vi "Calibrate_Sums_orig.vi"(8 "error in (no error)":errorcluster, 11 "Signal Channel":enum16{"Red", "Green"}(ring)) -> (0 "error out":errorcluster, 2 "sum":dbl)   [LabVIEW 2020]
doc: "Use this template to create a dialog box with event handling."
uses:
  Globals/gl_Calibration globals.vi
  Typedefs/Top level VI states.ctl
  Global Variables/gl_Images.vi
  Global Variables/General Globals.vi
  TypeDefs/Control Plane.ctl
panel:
  out "Objects found":T1(array[cluster])
  in  "Shape Adapted Options in":T2={"Number of Histogram Bins"=8, "Blending Parameter (%)"=10.0, "Max Scale Change (%)"=1.0, "Max Rotation Change"=40.0, "Max Shape Change (%)"=1.0, "Maximum Iterations"=15}
  out "Distance Array (Y)":dbl[][](array[numeric])
  in  "Delay 3":u32=1000
  out "Image 2":T3(plugin-control)
  out "Distance Array (X)":dbl[][](array[numeric])
  out "Image":T3(plugin-control)
  in  "Range":cluster{"Lower value":sgl, "Upper value":sgl}={"Lower value"=40.0, "Upper value"=255.0}
  in  "Delay 2":u32=1000
  in  "Delay":u32=1000
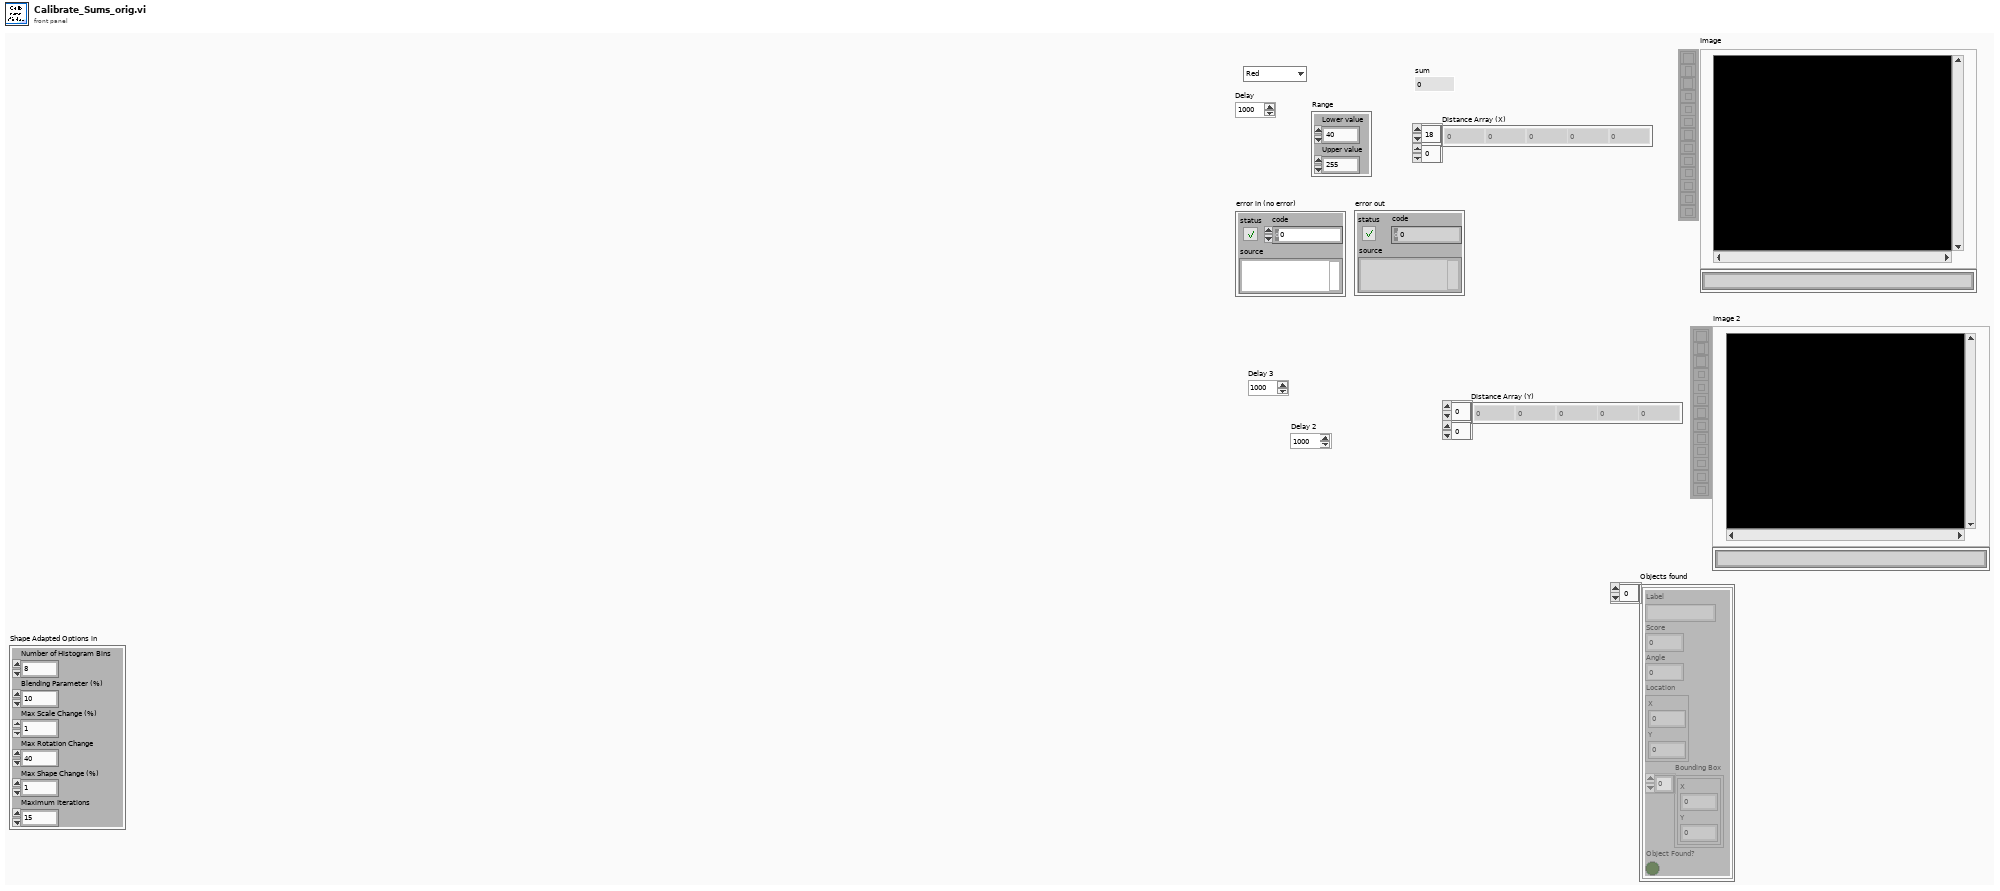
[diagram p1: front panel]
types:
  T1 = cluster{"Label":string, "Score":i32, "Angle":dbl, "Location":cluster{"X":dbl, "Y":dbl}, "Bounding Box":cluster{"X":dbl, "Y":dbl}[], "Object Found?":bool}[]
  T2 = cluster{"Number of Histogram Bins":i32, "Blending Parameter (%)":dbl, "Max Scale Change (%)":dbl, "Max Rotation Change":dbl, "Max Shape Change (%)":dbl, "Maximum Iterations":i32}
  T3 = typedef "IMAQ Image.ctl" = refnum<image>
  T4 = enum16{"Create tracking", "Setup Object", "Track Object", "Close"}
  T5 = enum16{"Raster", "Structural", "Pointing", "Mini Scan", "Alignment"}
  T6 = typedef "Top level VI states.ctl" = enum16{"None", "Initialise UI", "<STACK PROTOCOL STATES>", "AOL Zstack-START", "AOL Zstack-STOP", "Motor Zstack-START", "Motor Zstack-STOP", "<ACQUISITION PROTOCOL STATES> ", "Functional Acquisition-START", "Functional Acquisition-STOP", "Single Plane Acquisition-START", "Single Plane Acquisition-STOP", "Volume Acquisition-START", "Volume Acquisition-STOP", "<LIVE IMAGING PROTOCOL STATES>", "Live Imaging-START", "Live Imaging-STOP", "Live Plane Imaging-START", "Live Plane Imaging-STOP", "Live Volume Imaging-START", "Live Volume Imaging-STOP", "<MOVEMENT CORRECTION PROTOCOL STATES>", "EXIT"}
  T7 = typedef "Control Plane.ctl" = enum16{"XY-X", "XY-Y", "Z"}
  T8 = typedef "IMAQ Rectangle" = cluster{"Left":i32, "Top":i32, "Right":i32, "Bottom":i32, "Rotation":dbl}
  T9 = typedef "General Scan Parameters.ctl" = cluster{"Field of View":sgl, "Frame Size":u16, "Dwell Time (ms)":dbl, "Wavelength (nm)":dbl, "Zoom":dbl, "AOL Xc":sgl, "AOL Yc":sgl, "AOL Zc":sgl, "AOL Mode":enum16{"Raster", "Structural", "Pointing", "Mini Scan", "Alignment"}, "Imaging Mode":enum16{"Live Imaging", "AOL Zstack", "Motor Zstack", "Functional Imaging"}}
  T10 = cluster{"Particle Measurements (Pixels)[0]":dbl, "Particle Measurements (Pixels)[1]":dbl}[]
  T11 = typedef "Current Calibration Parameters.ctl" = cluster{"Sum X":dbl, "Sum Y":dbl, "Diff X":dbl, "Diff Y":dbl, "Distortion Correction":dbl, "Z_norm to um_scaling":dbl, "X_norm to um_scaling":dbl, "Samples to Wait after Trigger":dbl, "Slip Cycle":dbl}
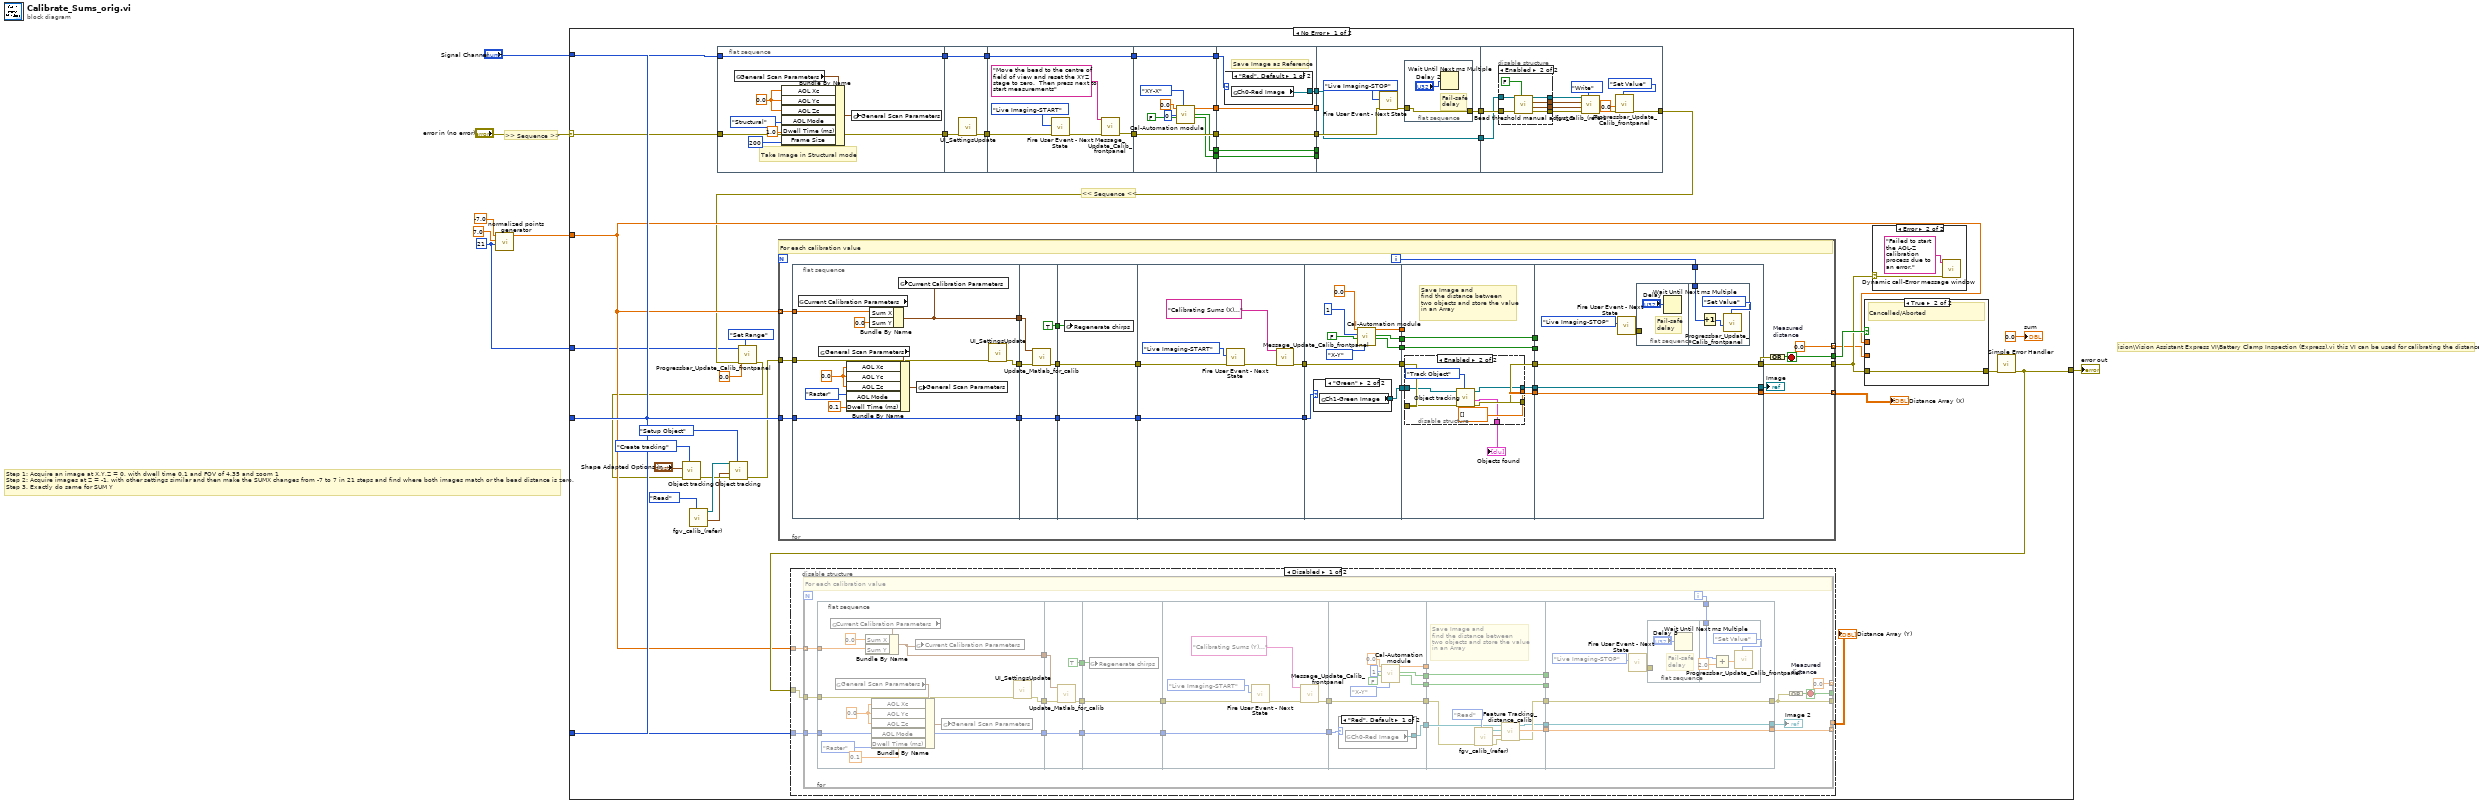
[diagram p0: block diagram]
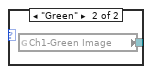
[diagram p2: hidden frame]
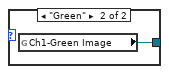
[diagram p4: hidden frame]
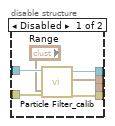
[diagram p5: hidden frame]
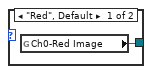
[diagram p6: hidden frame]
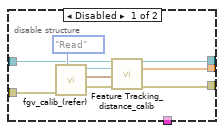
[diagram p7: hidden frame]
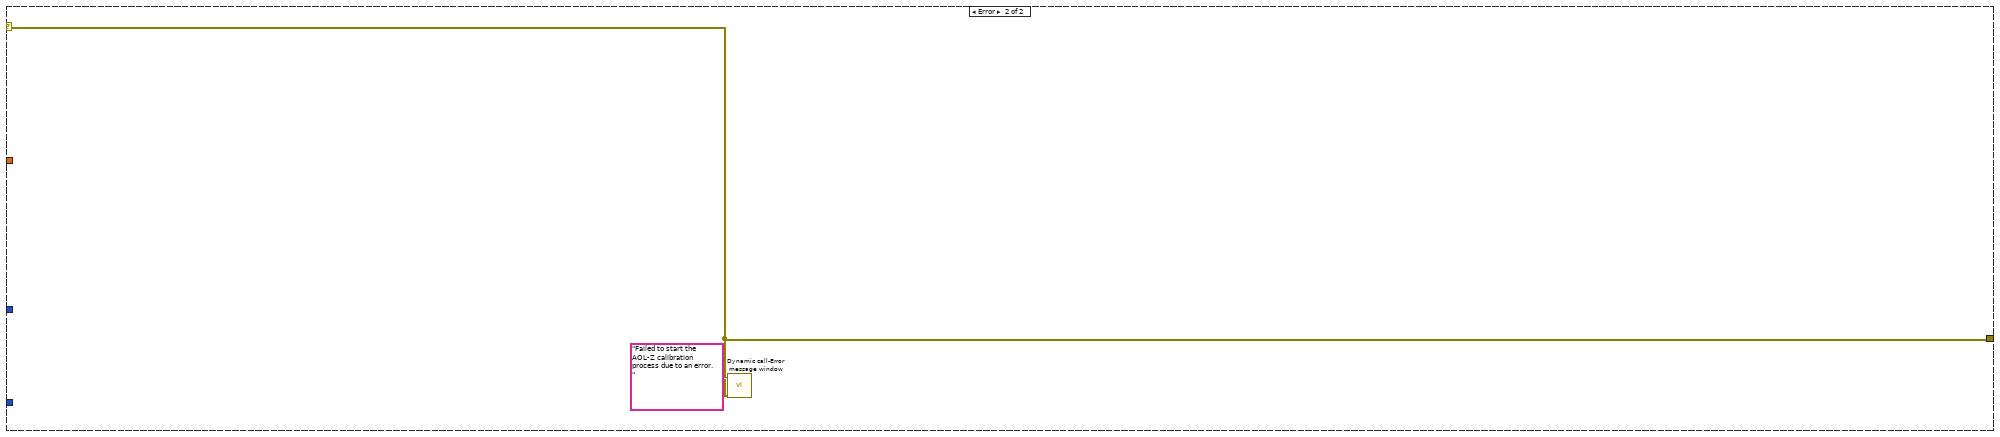
[diagram p10: hidden frame]
diagram:
  w1 = 21 ("number of points")
  # ">> Sequence >>"
  # "ision\\Vision Assistant Express VI\\Battery Clamp Inspection (Express).vi this VI can be used for calibrating the distance"
  # "Step 1: Acquire an image at X,Y,Z = 0, with dwell time 0.1 and FOV of 4.35 and zoom 1\nStep 2: Acquire images at Z = -1, with other settings similar and then make the SUMX changes from -7 to 7 in 21 steps and find where both images match or the bead distance is zero.\nStep 3. Exactly do same for SUM Y"
  n1 = call "normalized points generator.vi"("number of points"=w1, "maximum"=7.0, "minimum"=-7.0) -> ("normalised array"=w5:dbl[])  [unwired: 7 in, 1 out]
  n2 = case shown="No Error" "error in (no error)" {
    selector: "error in (no error)" -> [w45 w314]
    tunnel: w5 -> [w22 _]
    tunnel: [w23 w314] -> w7
    tunnel: "Signal Channel" -> [w27 _]
    tunnel: "Signal Channel" -> [w29 _]
    tunnel: "Signal Channel" -> [w24 _]
    tunnel: w1 -> [w17 _]
    frame No Error {
      # "<< Sequence <<"
      n3 = call "fgv_calib_(refer).vi"("State"=enum16{"Write", "Read"}."Read") -> ("enclosure box OUT"=w10:T8, "Reference Image"=w12:T3)  [unwired: 7 in, 2 out]
      n4 = flat-sequence {
        tunnel: w45 -> [w149]
        tunnel: [w149] -> w46
        tunnel: [w148] -> w30
        tunnel: w29 -> [w148]
        tunnel: [w155] -> w48
        tunnel: w46 -> [w154]
        tunnel: [w153] -> w31
        tunnel: w30 -> [w153]
        tunnel: [w160] -> w47
        tunnel: w48 -> [w161]
        tunnel: [w156] -> w32
        tunnel: w31 -> [w156]
        tunnel: [w169] -> w37
        tunnel: [w170] -> w39
        tunnel: w47 -> [w170]
        tunnel: [w165] -> w41
        tunnel: [w166] -> w43
        tunnel: [w163] -> w33
        tunnel: w32 -> [w163]
        tunnel: w43 -> [w176]
        tunnel: [w176] -> w42
        tunnel: w41 -> [w175]
        tunnel: [w175] -> w40
        tunnel: w39 -> [w174]
        tunnel: [w174] -> w38
        tunnel: w37 -> [w171]
        tunnel: [w171] -> w36
        tunnel: w33 -> [w173]
        tunnel: [w172] -> w28
        tunnel: w42 -> [_]
        tunnel: w40 -> [_]
        tunnel: w38 -> [w181]
        tunnel: w36 -> [_]
        tunnel: [w180] -> w35
        tunnel: w28 -> [w179]
        tunnel: [w179] -> w26
        tunnel: [w188] -> w18
        tunnel: w35 -> [w196]
        tunnel: w26 -> [w191]
        frame #0 {
          w150 = sgl 0.0 ("AOL Yc")
          # "Take Image in Structural mode"
          n5 = global read "gl_Calibration globals.vi" "General Scan Parameters"() -> (w152:T9)
          n6 = Bundle By Name(cluster=w152, "AOL Xc"=w150, "AOL Yc"=w150, "AOL Zc"=w150, "AOL Mode"=T5."Structural", "Dwell Time (ms)"=1.0, "Frame Size"=u16 200) -> (w151:T9)
          n7 = global write "gl_Calibration globals.vi" "General Scan Parameters"(w151) -> ()
        }
        frame #1 {
          n8 = call "UI_SettingsUpdate.vi"("error in (no error)"=w154) -> ("error out"=w155:errorcluster)  [unwired: 10 in]
        }
        frame #2 {
          n9 = call "Fire User Event - Next State.vi"("Error In"=w161, "\"UI Handler loop\" case to execute"=Top_level_VI_states."Live Imaging-START" ("\"UI Handler loop\" case to execute")) -> ("Error Out"=w159:errorcluster)  [unwired: 9 in]
          n10 = call "Message_Update_Calib_frontpanel.vi"("error in (no error)"=w159, "Message"="Move the bead to the centre of field of view and reset the XYZ stage to zero.  Then press next to start measurements") -> ("error out"=w160:errorcluster)  [unwired: 9 in]
        }
        frame #3 {
          n11 = call "Cal-Automation module.vi"("Parameter"=Control_Plane."XY-X", "Timed out while waiting for acknowledgement in"=FALSE, "FOR loop index"=0, "Initial motor position (um)"=sgl 0.0) -> ("Motor timed out or errored out"=w165:bool, "Cancelled"=w166:bool, "Measured cal value"=w169:sgl)  [unwired: 4 in, 1 out]
        }
        frame #4 {
          # "Save Image as Reference"
          n12 = case shown="\"Red\", Default" w173 {
            tunnel: [w177 w178] -> w172
            frame "Red", Default {
              n13 = global read "gl_Images.vi" "Ch0-Red Image"() -> (w177:T3)
            }
            frame "Green" {
              n14 = global read "gl_Images.vi" "Ch1-Green Image"() -> (w178:T3)
            }
          }
        }
        frame #5 {
          n15 = call "Fire User Event - Next State.vi"("Error In"=w181, "\"UI Handler loop\" case to execute"=Top_level_VI_states."Live Imaging-STOP" ("\"UI Handler loop\" case to execute")) -> ("Error Out"=w183:errorcluster)  [unwired: 9 in]
          n16 = flat-sequence {
            tunnel: w183 -> [w184]
            tunnel: [w184] -> w180
            frame #0 {
              # "Fail-safe delay"
              n17 = Wait Until Next ms Multiple(millisecond multiple="Delay 2") -> ()  [unwired: 1 out]
            }
          }
        }
        frame #6 {
          n18 = disable-structure shown="Enabled" {
            disable-tunnel: w196 -> [w202 w209]
            disable-tunnel: [w201 w206] -> w195
            disable-tunnel: [w200 w205] -> w194
            disable-tunnel: [w199 w204] -> w193
            disable-tunnel: w191 -> [w198 w208]
            disable-tunnel: [_ w203] -> w186
            frame Disabled {
              n19 = call "Particle Filter_calib.vi"("Range"="Range", "error in"=w202, "Source Image"=w198) -> ("error out"=w201:errorcluster, "Location in Pixels"=w199:T10, "Ref Image (8 bit)"=w200:T3)  [unwired: 6 in]
            }
            frame Enabled {
              n20 = call "Bead threshold manual adjust 2.vi"("Standalone(F)"=FALSE, "error in (no error)"=w209, "Image In"=w208) -> ("error out"=w206:errorcluster, "enclosure box"=w203:T8, "Centroid array"=w204:T10, "Source Image"=w205:T3)  [unwired: 4 in]
            }
          }
          n21 = call "fgv_calib_(refer).vi"("State"=enum16{"Write", "Read"}."Write", "error in (no error)"=w195, "enclosure box IN"=w186, "Location in Pixels"=w193, "Reference Image"=w194) -> ("error in (no error)"=w189:errorcluster)  [unwired: 3 in, 3 out]
          n22 = call "Progressbar_Update_Calib_frontpanel.vi"("Ops"=enum16{"Set Value", "Set Range"}."Set Value", "error in (no error)"=w189, "Value"=0.0) -> ("error out"=w188:errorcluster)  [unwired: 8 in]
        }
      }
      n23 = call "Progressbar_Update_Calib_frontpanel.vi"("Ops"=enum16{"Set Value", "Set Range"}."Set Range", "error in (no error)"=w18, "Scale.Range:Minimum"=0.0, "Scale.Range:Maximum"=w17) -> ("error out"=w9:errorcluster)  [unwired: 7 in]
      n24 = call "Object tracking.vi"("Tracking Ops"=T4."Create tracking", "error in (no error)"=w9, "Shape Adapted Options in"="Shape Adapted Options in") -> ("error out"=w11:errorcluster)  [unwired: 2 in, 6 out]
      n25 = call "Object tracking.vi"("Tracking Ops"=T4."Setup Object", "error in (no error)"=w11, "Rectangle"=w10, "Image IN"=w12) -> ("error out"=w8:errorcluster)  [unwired: 1 in, 6 out]
      n26 = for {
        tunnel: w22 -> [w238] mode=indexing
        tunnel: [w233] -> w50
        tunnel: [w234] -> w49
        tunnel: w8 -> [w236]
        tunnel: [w224] -> w44 mode=indexing
        tunnel: w27 -> [w223]
        tunnel: [w218] -> w25 mode=indexing
        i -> [w210]
        stop <- w233 stop-if-true
        w224 = sgl 0.0  # Measured  distance
        # "For each calibration value"
        n27 = flat-sequence {
          tunnel: w238 -> [w249]
          tunnel: w236 -> [w240]
          tunnel: [w239] -> w235
          tunnel: [w248] -> w225
          tunnel: w223 -> [w246]
          tunnel: [w246] -> w222
          tunnel: w235 -> [w255]
          tunnel: [w254] -> w217
          tunnel: w225 -> [w253]
          tunnel: w222 -> [w252]
          tunnel: [w252] -> w215
          tunnel: [TRUE] -> w213
          tunnel: w217 -> [w258]
          tunnel: [w258] -> w216
          tunnel: w215 -> [w257]
          tunnel: [w257] -> w214
          tunnel: w213 -> [w256]
          tunnel: [w263] -> w237
          tunnel: w216 -> [w264]
          tunnel: w214 -> [w259]
          tunnel: [w259] -> w221
          tunnel: [w273] -> w232
          tunnel: [w274] -> w231
          tunnel: w237 -> [w274]
          tunnel: [w269] -> w229
          tunnel: [w270] -> w227
          tunnel: w221 -> [w265]
          tunnel: [w266] -> w220
          tunnel: w232 -> [_]
          tunnel: w231 -> [w280]
          tunnel: [w279] -> w230
          tunnel: w229 -> [w284]
          tunnel: [w284] -> w228
          tunnel: w227 -> [w283]
          tunnel: [w283] -> w226
          tunnel: w220 -> [w282]
          tunnel: [w281] -> w219
          tunnel: [w278] -> w212
          tunnel: w230 -> [w305]
          tunnel: [w305] -> w234
          tunnel: w228 -> [_]
          tunnel: w226 -> [_]
          tunnel: w219 -> [w303]
          tunnel: [w303] -> w218
          tunnel: [w302] -> w211
          tunnel: w212 -> [w302]
          tunnel: w210 -> [w301]
          frame #0 {
            w243 = sgl 0.0 ("AOL Yc")
            n28 = global read "gl_Calibration globals.vi" "Current Calibration Parameters"() -> (w250:T11)
            n29 = global read "gl_Calibration globals.vi" "General Scan Parameters"() -> (w245:T9)
            n30 = Bundle By Name(cluster=w245, "AOL Xc"=w243, "AOL Yc"=w243, "AOL Zc"=w243, "AOL Mode"=T5."Raster", "Dwell Time (ms)"=0.1) -> (w244:T9)
            n31 = Bundle By Name(cluster=w250, "Sum X"=w249, "Sum Y"=0.0) -> (w248:T11)
            n32 = global write "gl_Calibration globals.vi" "Current Calibration Parameters"(w248) -> ()
            n33 = global write "gl_Calibration globals.vi" "General Scan Parameters"(w244) -> ()
            n34 = call "UI_SettingsUpdate.vi"("error in (no error)"=w240) -> ("error out"=w239:errorcluster)  [unwired: 10 in]
          }
          frame #1 {
            n35 = call "Update_Matlab_for_calib.vi"("error in (no error)"=w255, "Current Calibration Parameters"=w253) -> ("error out"=w254:errorcluster)  [unwired: 9 in]
          }
          frame #2 {
            n36 = global write "General Globals.vi" "Regenerate chirps"(w256) -> ()
          }
          frame #3 {
            n37 = call "Fire User Event - Next State.vi"("Error In"=w264, "\"UI Handler loop\" case to execute"=Top_level_VI_states."Live Imaging-START" ("\"UI Handler loop\" case to execute")) -> ("Error Out"=w262:errorcluster)  [unwired: 9 in]
            n38 = call "Message_Update_Calib_frontpanel.vi"("error in (no error)"=w262, "Message"="Calibrating Sums (X)...") -> ("error out"=w263:errorcluster)  [unwired: 9 in]
          }
          frame #4 {
            n39 = case shown="\"Green\"" w265 {
              tunnel: [w275 w276] -> w266
              frame "Red", Default {
                n40 = global read "gl_Images.vi" "Ch0-Red Image"() -> (w275:T3)
              }
              frame "Green" {
                n41 = global read "gl_Images.vi" "Ch1-Green Image"() -> (w276:T3)
              }
            }
            n42 = call "Cal-Automation module.vi"(6:enum16{"X-Y", "Z"}."X-Y" ("StageSelection"), "Timed out while waiting for acknowledgement in"=FALSE, "FOR loop index"=1, "Initial motor position (um)"=sgl 0.0) -> ("Motor timed out or errored out"=w269:bool, "Cancelled"=w270:bool, "Measured cal value"=w273:sgl)  [unwired: 4 in, 1 out]
          }
          frame #5 {
            # "Save Image and \nfind the distance between\ntwo objects and store the value\nin an Array"
            n43 = disable-structure shown="Enabled" {
              disable-tunnel: w282 -> [w290 w299]
              disable-tunnel: [w289 dbl[] [] ("Distance Array")] -> w281
              disable-tunnel: w280 -> [w287 w300]
              disable-tunnel: [w286 w295] -> w279
              disable-tunnel: [w285 w296] -> w278
              disable-tunnel: [_ w294] -> w277
              frame Disabled {
                n44 = call "fgv_calib_(refer).vi"("State"=enum16{"Write", "Read"}."Read", "error in (no error)"=w287) -> ("error in (no error)"=w288:errorcluster, "Location in Pixels"=w291:T10, "Reference Image"=w292:T3)  [unwired: 6 in, 1 out]
                n45 = call "Feature Tracking_distance_calib.vi"("Current Image"=w290, "Reference Image"=w292, "Location in Pixels"=w291, "error in (no error)"=w288) -> ("Analysed Image"=w285:T3, "Distance Array"=w289:dbl[], "error out"=w286:errorcluster)  [unwired: 9 in]
              }
              frame Enabled {
                n46 = call "Object tracking.vi"("Tracking Ops"=T4."Track Object", "error in (no error)"=w300, "Image IN"=w299) -> ("error out"=w295:errorcluster, "Objects found"=w294:T1, "Image OUT"=w296:T3)  [unwired: 2 in, 4 out]
              }
            }
            "Objects found" <- w277
          }
          frame #6 {
            n47 = call "Fire User Event - Next State.vi"("\"UI Handler loop\" case to execute"=Top_level_VI_states."Live Imaging-STOP" ("\"UI Handler loop\" case to execute")) -> ("Error Out"=w306:errorcluster)  [unwired: 10 in]
            n48 = flat-sequence {
              tunnel: w306 -> [_]
              tunnel: w301 -> [w309]
              frame #0 {
                # "Fail-safe delay"
                n49 = Wait Until Next ms Multiple(millisecond multiple="Delay") -> ()  [unwired: 1 out]
              }
              frame #1 {
                n50 = Increment(x=w309) -> (x+1=w308:i32)
                n51 = call "Progressbar_Update_Calib_frontpanel.vi"("Ops"=enum16{"Set Value", "Set Range"}."Set Value", "Value"=w308) -> ()  [unwired: 9 in, 1 out]
              }
            }
          }
        }
        n52 = Compound Arithmetic op=OR(w234) -> (w233:bool)
        "Image" <- w211
      }
      "Distance Array (X)" <- w25
      n53 = case shown="True" w50 {
        tunnel: w22 -> [_ _]
        tunnel: w44 -> [_ _]
        tunnel: [_ w313] -> w51
        tunnel: w49 -> [_ w313]
        frame False {
          # "find zero value from the array"
        }
        frame True {
          # "Cancelled/Aborted"
        }
      }
      n54 = case shown="Error" w49 {
        selector: w49 -> [_ w312]
        frame No Error {
        }
        frame Error {
          n55 = call "Dynamic call-Error message window.vi"("error in (no error)"=w312, "Error Message"="Failed to start the AOL-Z calibration process due to an error.") -> ()  [unwired: 9 in, 1 out]
        }
      }
      n56 = call <vilib>:"Simple Error Handler.vi"("error in (no error)"=w51) -> ("error out"=w23:errorcluster)  [unwired: 4 in, 4 out]
      n57 = disable-structure shown="Disabled" {
        disable-tunnel: w24 -> [w55 _]
        disable-tunnel: w23 -> [w54 _]
        disable-tunnel: w22 -> [w53 _]
        disable-tunnel: [w52 _] -> w21
        frame Disabled {
          n58 = for {
            tunnel: w53 -> [w84] mode=indexing
            tunnel: [w79] -> _
            tunnel: [w80] -> _
            tunnel: w54 -> [w82]
            tunnel: [w70] -> _ mode=indexing
            tunnel: w55 -> [w69]
            tunnel: [w64] -> w52 mode=indexing
            i -> [w56]
            stop <- w79 stop-if-true
            w70 = sgl 0.0  # Measured  distance
            # "For each calibration value"
            n59 = flat-sequence {
              tunnel: w84 -> [w85]
              tunnel: w82 -> [w88]
              tunnel: [w87] -> w81
              tunnel: [w95] -> w71
              tunnel: w69 -> [w94]
              tunnel: [w94] -> w68
              tunnel: w81 -> [w101]
              tunnel: [w100] -> w63
              tunnel: w71 -> [w99]
              tunnel: w68 -> [w98]
              tunnel: [w98] -> w61
              tunnel: [TRUE] -> w59
              tunnel: w63 -> [w104]
              tunnel: [w104] -> w62
              tunnel: w61 -> [w103]
              tunnel: [w103] -> w60
              tunnel: w59 -> [w102]
              tunnel: [w109] -> w83
              tunnel: w62 -> [w110]
              tunnel: w60 -> [w105]
              tunnel: [w105] -> w67
              tunnel: [w119] -> w78
              tunnel: [w120] -> w77
              tunnel: w83 -> [w120]
              tunnel: [w115] -> w75
              tunnel: [w116] -> w73
              tunnel: w67 -> [w111]
              tunnel: [w112] -> w66
              tunnel: w78 -> [_]
              tunnel: w77 -> [w125]
              tunnel: [w124] -> w76
              tunnel: w75 -> [w133]
              tunnel: [w133] -> w74
              tunnel: w73 -> [w132]
              tunnel: [w132] -> w72
              tunnel: w66 -> [w128]
              tunnel: [w127] -> w65
              tunnel: [w123] -> w58
              tunnel: w76 -> [w138]
              tunnel: [w138] -> w80
              tunnel: w74 -> [_]
              tunnel: w72 -> [_]
              tunnel: w65 -> [w136]
              tunnel: [w136] -> w64
              tunnel: [w135] -> w57
              tunnel: w58 -> [w135]
              tunnel: w56 -> [w134]
              frame #0 {
                w91 = sgl 0.0 ("AOL Yc")
                n60 = global read "gl_Calibration globals.vi" "Current Calibration Parameters"() -> (w96:T11)
                n61 = global read "gl_Calibration globals.vi" "General Scan Parameters"() -> (w93:T9)
                n62 = Bundle By Name(cluster=w96, "Sum X"=0.0 ("Sum Y"), "Sum Y"=w85) -> (w95:T11)
                n63 = Bundle By Name(cluster=w93, "AOL Xc"=w91, "AOL Yc"=w91, "AOL Zc"=w91, "AOL Mode"=T5."Raster", "Dwell Time (ms)"=0.1) -> (w92:T9)
                n64 = global write "gl_Calibration globals.vi" "Current Calibration Parameters"(w95) -> ()
                n65 = global write "gl_Calibration globals.vi" "General Scan Parameters"(w92) -> ()
                n66 = call "UI_SettingsUpdate.vi"("error in (no error)"=w88) -> ("error out"=w87:errorcluster)  [unwired: 10 in]
              }
              frame #1 {
                n67 = call "Update_Matlab_for_calib.vi"("error in (no error)"=w101, "Current Calibration Parameters"=w99) -> ("error out"=w100:errorcluster)  [unwired: 9 in]
              }
              frame #2 {
                n68 = global write "General Globals.vi" "Regenerate chirps"(w102) -> ()
              }
              frame #3 {
                n69 = call "Fire User Event - Next State.vi"("Error In"=w110, "\"UI Handler loop\" case to execute"=Top_level_VI_states."Live Imaging-START" ("\"UI Handler loop\" case to execute")) -> ("Error Out"=w108:errorcluster)  [unwired: 9 in]
                n70 = call "Message_Update_Calib_frontpanel.vi"("error in (no error)"=w108, "Message"="Calibrating Sums (Y)...") -> ("error out"=w109:errorcluster)  [unwired: 9 in]
              }
              frame #4 {
                n71 = case shown="\"Red\", Default" w111 {
                  tunnel: [w121 w122] -> w112
                  frame "Red", Default {
                    n72 = global read "gl_Images.vi" "Ch0-Red Image"() -> (w121:T3)
                  }
                  frame "Green" {
                    n73 = global read "gl_Images.vi" "Ch1-Green Image"() -> (w122:T3)
                  }
                }
                n74 = call "Cal-Automation module.vi"(6:enum16{"X-Y", "Z"}."X-Y" ("StageSelection"), "Timed out while waiting for acknowledgement in"=FALSE, "FOR loop index"=1, "Initial motor position (um)"=sgl 0.0) -> ("Motor timed out or errored out"=w115:bool, "Cancelled"=w116:bool, "Measured cal value"=w119:sgl)  [unwired: 4 in, 1 out]
              }
              frame #5 {
                # "Save Image and \nfind the distance between\ntwo objects and store the value\nin an Array"
                n75 = call "fgv_calib_(refer).vi"("State"=enum16{"Write", "Read"}."Read", "error in (no error)"=w125) -> ("error in (no error)"=w126:errorcluster, "Location in Pixels"=w129:T10, "Reference Image"=w130:T3)  [unwired: 6 in, 1 out]
                n76 = call "Feature Tracking_distance_calib.vi"("error in (no error)"=w126, "Location in Pixels"=w129, "Reference Image"=w130, "Current Image"=w128) -> ("error out"=w124:errorcluster, "Distance Array"=w127:dbl[], "Analysed Image"=w123:T3)  [unwired: 5 in]
              }
              frame #6 {
                n77 = call "Fire User Event - Next State.vi"("\"UI Handler loop\" case to execute"=Top_level_VI_states."Live Imaging-STOP" ("\"UI Handler loop\" case to execute")) -> ("Error Out"=w139:errorcluster)  [unwired: 10 in]
                n78 = flat-sequence {
                  tunnel: w139 -> [_]
                  tunnel: w134 -> [w141]
                  frame #0 {
                    # "Fail-safe delay"
                    n79 = Wait Until Next ms Multiple(millisecond multiple="Delay 3") -> ()  [unwired: 1 out]
                  }
                  frame #1 {
                    n80 = Add(x=w141, y=2.0) -> (x+y=w142:dbl)
                    n81 = call "Progressbar_Update_Calib_frontpanel.vi"("Ops"=enum16{"Set Value", "Set Range"}."Set Value", "Value"=w142) -> ()  [unwired: 9 in, 1 out]
                  }
                }
              }
            }
            n82 = Compound Arithmetic op=OR(w80) -> (w79:bool)
            "Image 2" <- w57
          }
        }
        frame Enabled {
        }
      }
      "Distance Array (Y)" <- w21
      "sum" <- 0.0 ("sum")
    }
    frame Error {
      n83 = call "Dynamic call-Error message window.vi"("error in (no error)"=w314, "Error Message"="Failed to start the AOL-Z calibration process due to an error.") -> ()  [unwired: 9 in, 1 out]
    }
  }
  "error out" <- w7
